vi "File_ExistsFile.vi"(11 "Value":path) -> (0 "error out":errorcluster, 2 "Boolean":bool, 3 "dup path":path)   [LabVIEW 2016]
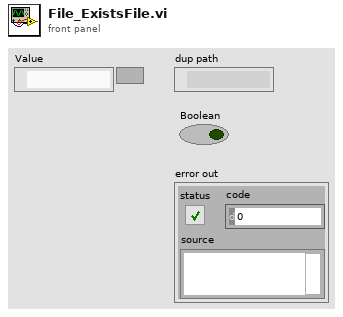
[diagram p1: front panel]
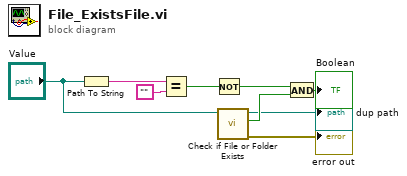
[diagram p0: block diagram]
diagram:
  n1 = Path To String(path="Value") -> (string=w5:string)
  n2 = Equal?(x=w5, y="") -> (x = y?=w8:bool)
  n3 = Not(x=w8) -> (.not. x?=w9:bool)
  n4 = call <vilib>:"Check if File or Folder Exists.vi"("path"="Value") -> ("error out"=→"error out":errorcluster, "file or folder exists?"=w3:bool, "dup path"=→"dup path":path)  [unwired: 8 in]
  n5 = And(x=w9, y=w3) -> (x .and. y?=→"Boolean":bool)
